vi "main.vi"() -> ()   [LabVIEW 2015, in "lv-example-postgres-post-installer.lvlib"]
uses:
  lv-example-postgres-post-installer.lvlib
  <userlib>/antonio-alexander/lv-post-installer/lv-post-installer/public/classes/lv-post-installer/lv-post-installer.lvclass
  odbc_driver_postgres_v13.0.2/odbc_driver_postgres_v13.0.2.lvclass
  <userlib>/antonio-alexander/lv-post-installer/lv-post-installer-interface/lv-post-installer-interface.lvlib
panel:
  out "error":errorcluster
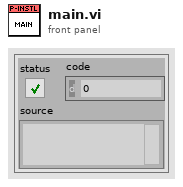
[diagram p1: front panel]
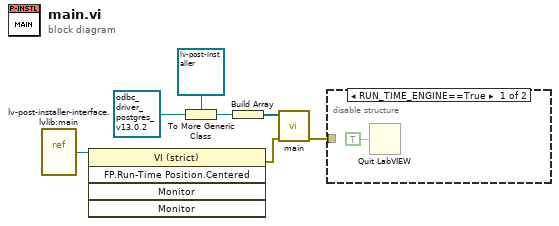
[diagram p0: block diagram]
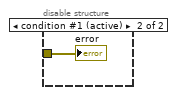
[diagram p2: hidden frame]
diagram:
  n1 = vi-ref "lv-post-installer-interface.lvlib:main.vi"() -> (w4:refnum<vi>)
  n2 = invoke class="VI (strict)" method="FP.Run-Time Position.Centered"(reference=w4) -> (error out=w3:errorcluster)  [unwired: 4 in, 4 out]
  n3 = To More Generic Class(target class=refnum<class "lv-post-installer.lvclass"> refnum ("lv-post-installer.lvlib:lv-post-installer.lvclass"), reference=refnum<class "odbc_driver_postgres_v13.0.2.lvclass"> refnum ("lv-timescaledb-post-installer.lvlib:odbc_driver_postgres_v13.0.2.lvclass")) -> (generic class reference=w7:refnum<class "lv-post-installer.lvclass">)
  n4 = Build Array(w7) -> (w1:refnum<class "lv-post-installer.lvclass">[])
  n5 = call <userlib>:"main.vi"("error in (no error)"=w3, "post_installer []"=w1) -> ("error out"=w2:errorcluster)  [unwired: 9 in]
  n6 = disable-structure shown="RUN_TIME_ENGINE==True" {
    disable-tunnel: w2 -> [_ w9]
    frame condition #0 {
      n7 = Quit LabVIEW(quit? (T)=TRUE) -> ()
    }
    frame condition #1 (active) {
      "error" <- w9
    }
  }
